vi "serialPlot3Ax (1).vi"() -> ()   [LabVIEW 2017]
uses:
  <vilib>/Utility/error.llb/DialogType.ctl
  <vilib>/Instr/_visa.llb/VISA Configure Serial Port (Instr).vi
  <vilib>/ptbypt/NI_PtbyPt.lvlib
panel:
  out "Elapsed Time (s)":dbl
  in  "Time":dbl
  out "Mean":dbl format="%#.6f"
  out "Mean":dbl format="%#.7f"
  out "Y axis":i32(graph)
  out "Z Axis":i32(graph)
  out "Mean":dbl format="%#.7f"
  out "X axis":i32(graph)
  in  "1 Axis":bool caption="3 Axes"
  out "?":bool
  in  "Record":bool
  in  "Baud Rate":u32(ring)=115200 items=["75"=75, "110"=110, "134"=134, "150"=150, "300"=300, "600"=600, "1200"=1200, "1800"=1800, "2400"=2400, "4800"=4800, "7200"=7200, "9600"=9600, "14400"=14400, "19200"=19200, "28800"=28800, "38400"=38400, "56000"=56000, "57600"=57600, "115200"=115200, "128000"=128000, "230400"=230400]
  in  "Stop":bool
  in  "Port":refnum<visa-resource-name>
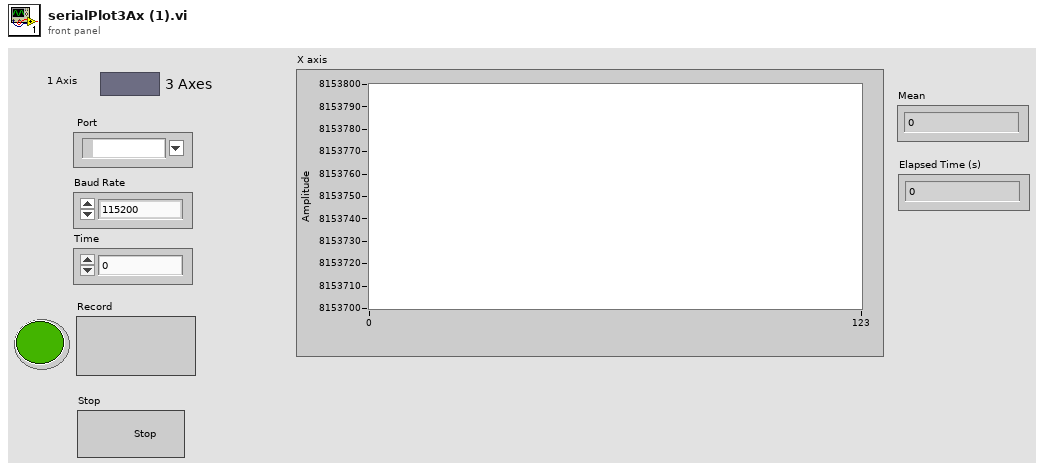
[diagram p1: front panel]
types:
  T1 = typedef "DialogType.ctl" = u16
  T2 = enum16{"open", "replace", "create", "open or create", "replace or create", "replace or create with confirmation"}
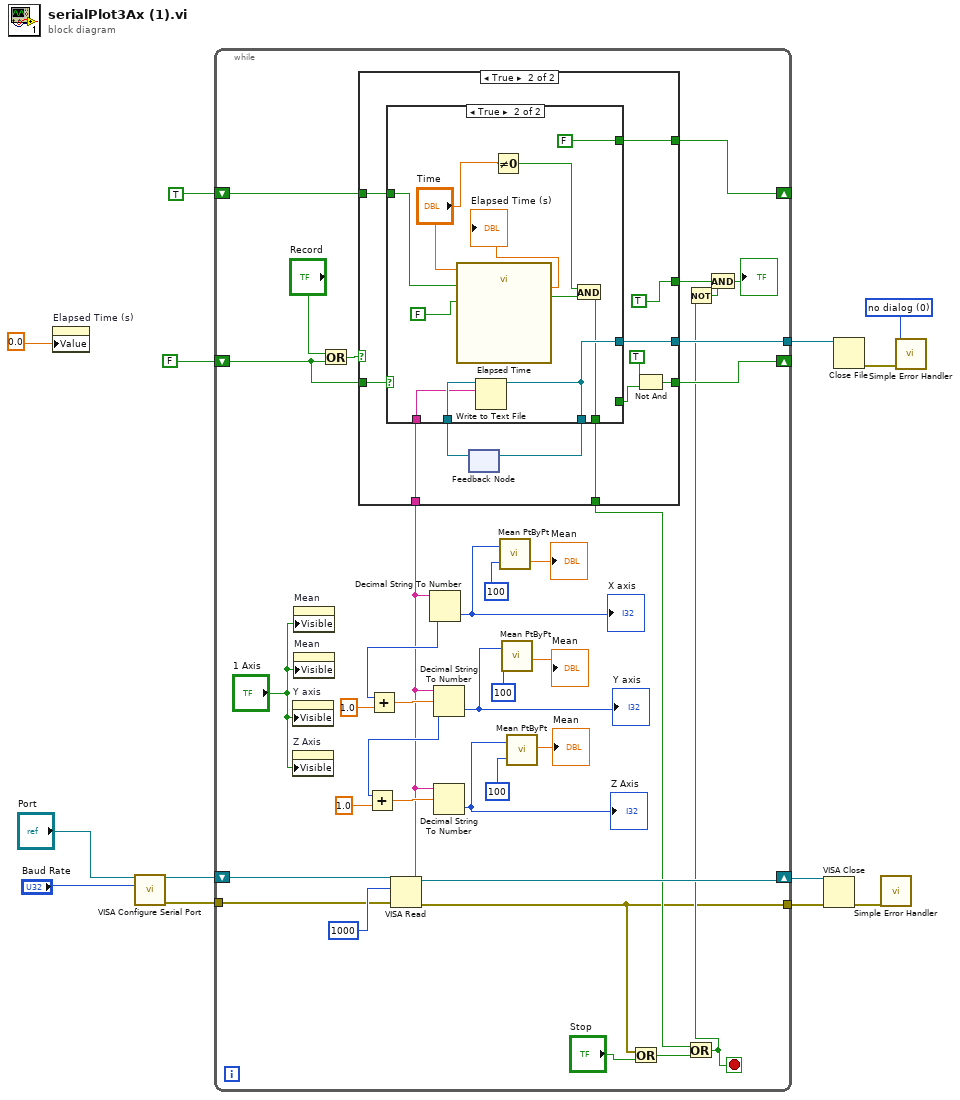
[diagram p0: block diagram]
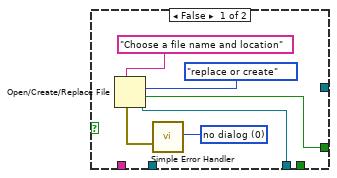
[diagram p3: hidden frame]
diagram:
  w4 = T1 0 items=["no dialog", "OK message", "continue or stop message", "OK message + warnings", "continue/stop + warnings"] ("type of dialog (OK msg:1)")
  n1 = property on="Elapsed Time (s)" class="DigNum (strict)"("Value"=0.0 ("Elapsed Time (s)")) -> ()  [unwired: 2 in, 2 out]
  n2 = call-poly "VISA Configure Serial Port"("VISA resource name"="Port", "baud rate (9600)"="Baud Rate") -> ("VISA resource name out"=w12:refnum<visa-resource-name>, "error out"=w11:errorcluster)  [unwired: 12 in]
  n3 = while {
    tunnel: w11 -> [w43]
    shift-right: [w47] -> w10
    shift-left: w12 -> [w49]
    tunnel: [w18] -> w9
    shift-right: [w44] -> _
    shift-left: FALSE ("x") -> [w15]
    tunnel: [w42] -> w6
    shift-right: [w16] -> _
    shift-left: TRUE -> [w14]
    stop <- w39 stop-if-true
    n4 = property on="Y axis" class="WFChart (strict)"("Visible"="1 Axis") -> ()  [unwired: 2 in, 2 out]
    n5 = property on="Z Axis" class="WFChart (strict)"("Visible"="1 Axis") -> ()  [unwired: 2 in, 2 out]
    n6 = property on="Mean" class="DigNum (strict)"("Visible"="1 Axis") -> ()  [unwired: 2 in, 2 out]
    n7 = property on="Mean" class="DigNum (strict)"("Visible"="1 Axis") -> ()  [unwired: 2 in, 2 out]
    n8 = Or(x="Record", y=w15) -> (x .or. y?=w46:bool)
    n9 = VISA Read(VISA resource name=w49, byte count=u32 1000, error in (no error)=w43) -> (VISA resource name out=w47:refnum<visa-resource-name>, read buffer=w22:string, error out=w18:errorcluster)  [unwired: 1 out]
    n10 = case shown="True" w46 {
      tunnel: w15 -> [w50 w54]
      tunnel: [w50 w57] -> w44
      tunnel: w22 -> [_ w60]
      tunnel: [_ w59] -> w42
      tunnel: [_ TRUE] -> w41
      tunnel: [_ w53] -> w20
      tunnel: w14 -> [_ w52]
      tunnel: [_ w51] -> w16
      frame False {
      }
      frame True {
        n11 = feedback #1() -> (w61:refnum<file>)  [unwired: 1 in]
        n12 = case shown="True" w54 {
          tunnel: [w67 w77] -> w62
          tunnel: w61 -> [_ w79]
          tunnel: w60 -> [_ w78]
          tunnel: [_ w77] -> w59
          tunnel: [w65 _] -> w58
          tunnel: [_ w69] -> w53
          tunnel: w52 -> [_ w75]
          tunnel: [_ FALSE] -> w51
          frame False {
            w63 = T1 0 items=["no dialog", "OK message", "continue or stop message", "OK message + warnings", "continue/stop + warnings"] ("type of dialog (OK msg:1)")
            n13 = Open/Create/Replace File(prompt="Choose a file name and location", operation (0:open)=T2."replace or create") -> (refnum out=w67:refnum<file>, cancelled=w65:bool, error out=w64:errorcluster)  [unwired: 4 in]
            n14 = call <vilib>:"Simple Error Handler.vi"("type of dialog (OK msg:1)"=w63, "error in (no error)"=w64) -> ()  [unwired: 3 in, 5 out]
          }
          frame True {
            n15 = call "Elapsed Time"("Time Target (s)"="Time", "Reset"=w75, "Auto Reset"=FALSE) -> ("Elapsed Time (s)"=→"Elapsed Time (s)":dbl, "Time has Elapsed"=w71:bool)  [unwired: 9 in, 6 out]
            n16 = Write to Text File(file (use dialog)=w79, text=w78) -> (refnum out=w77:refnum<file>)  [unwired: 2 in, 2 out]
            n17 = Not Equal To 0?(x="Time") -> (x != 0?=w70:bool)
            n18 = And(x=w70, y=w71) -> (x .and. y?=w69:bool)
          }
        }
        n19 = feedback-in #1(w62) -> ()
        n20 = Not And(1:w58, 2:TRUE) -> (0:w57:bool)
      }
    }
    n21 = Decimal String To Number(string=w22) -> (offset past number=w24:i32, number=w23:i32)  [unwired: 2 in]
    "X axis" <- w23
    n22 = Add(x=w24, y=1.0) -> (x+y=w35:dbl)
    n23 = Decimal String To Number(string=w22, offset=w35) -> (offset past number=w31:i32, number=w29:i32)  [unwired: 1 in]
    "Y axis" <- w29
    n24 = Add(x=w31, y=1.0) -> (x+y=w32:dbl)
    n25 = Decimal String To Number(string=w22, offset=w32) -> (number=w25:i32)  [unwired: 1 in, 1 out]
    "Z Axis" <- w25
    n26 = call <vilib>:"Mean PtByPt.vi"("x"=w23, "sample length"=100) -> ("mean"=→"Mean":dbl)  [unwired: 2 in, 1 out]
    n27 = call <vilib>:"Mean PtByPt.vi"("x"=w29, "sample length"=100) -> ("mean"=→"Mean":dbl)  [unwired: 2 in, 1 out]
    n28 = call <vilib>:"Mean PtByPt.vi"("x"=w25, "sample length"=100) -> ("mean"=→"Mean":dbl)  [unwired: 2 in, 1 out]
    n29 = Or(x=w18, y="Stop") -> (x .or. y?=w17:bool)
    n30 = Or(x=w20, y=w17) -> (x .or. y?=w39:bool)
    n31 = Not(x=w39) -> (.not. x?=w40:bool)
    n32 = And(x=w41, y=w40) -> (x .and. y?=→"?":bool)
  }
  n33 = VISA Close(VISA resource name=w10, error in (no error)=w9) -> (error out=w8:errorcluster)
  n34 = Close File(refnum=w6) -> (error out=w5:errorcluster)  [unwired: 1 in, 1 out]
  n35 = call <vilib>:"Simple Error Handler.vi"("error in (no error)"=w8) -> ()  [unwired: 4 in, 5 out]
  n36 = call <vilib>:"Simple Error Handler.vi"("type of dialog (OK msg:1)"=w4, "error in (no error)"=w5) -> ()  [unwired: 3 in, 5 out]
